vi "Green Board DC Bus Test.vi"(7 "HMP4040 Channel Settings":T1={"CH1 Voltage"=24.0, "CH1 Current"=1.0, "CH1 Output"=FALSE, "CH2 Voltage"=24.0, "CH2 Current"=3.0, "CH2 Output"=TRUE, "CH3 Voltage"=24.0, "CH3 Current"=1.0, "CH3 Output"=FALSE, "CH4 Voltage"=24.0, "CH4 Current"=1.0, "CH4 Output"=FALSE, "Master Output"=TRUE} {"CH4 Current" format="%.3f"; "CH4 Voltage" format="%.3f"; "CH3 Current" format="%.3f"; "CH3 Voltage" format="%.3f"; "CH2 Current" format="%.3f"; "CH2 Voltage" format="%.3f"; "CH1 Current" format="%.3f"; "CH1 Voltage" format="%.3f"}, 8 "error in (no error)":errorcluster, 9 "Board Selector":T2) -> (0 "error out":errorcluster, 2 "Message OUT":string, 3 "VISA Refnum out":refnum<visa-resource-name>, 5 "Pass/Fail":bool, 10 "Voltage DC charged":dbl, 11 "Voltage (0V)":dbl)   [LabVIEW 2022 SP3]
uses:
  Serial Board Com/Board Select.ctl
  HMP4000 Communication/HMP4040_ChannelControl.ctl
  Serial Board Com/ADCSelector GB.ctl
panel:
  in  "Message IN":string
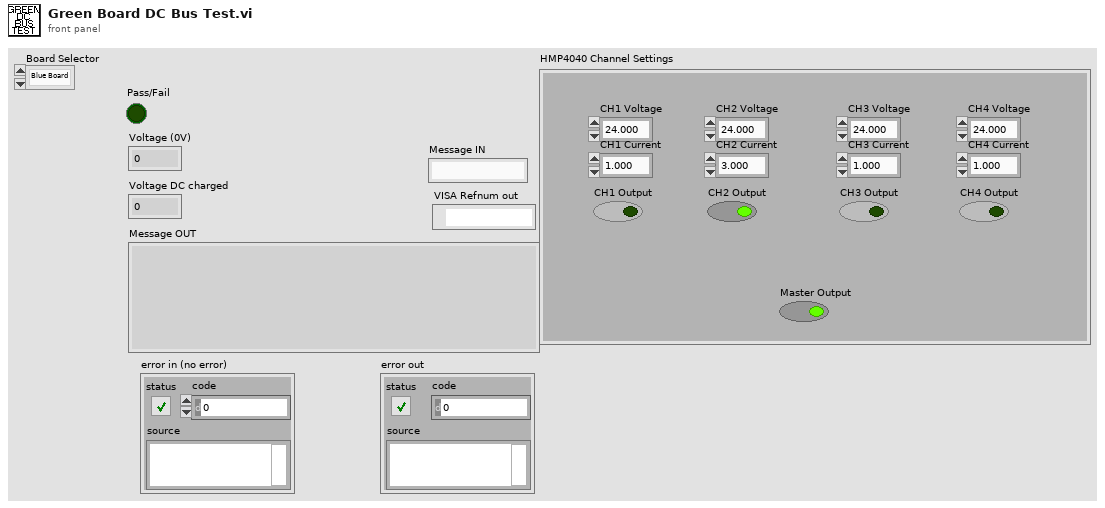
[diagram p1: front panel]
types:
  T1 = typedef "HMP4040_ChannelControl.ctl" = cluster{"CH1 Voltage":dbl, "CH1 Current":dbl, "CH1 Output":bool, "CH2 Voltage":dbl, "CH2 Current":dbl, "CH2 Output":bool, "CH3 Voltage":dbl, "CH3 Current":dbl, "CH3 Output":bool, "CH4 Voltage":dbl, "CH4 Current":dbl, "CH4 Output":bool, "Master Output":bool}
  T2 = typedef "Board Select.ctl" = enum16{"Blue Board", "Green Board"}
  T3 = typedef "ADCSelector GB.ctl" = enum16{"INVA_ISENSE_U", "INVA_ISENSE_V", "INVA_ISENSE_W", "INVA_UDC", "INVA_TEMP", "HB_ISENSE", "AUX_ISENSE_U", "AUX_ISENSE_V", "AUX_ISENSE_W", "VLINE_AB", "VLINE_BC", "VLINE_CA", "REF_1P5V", "VSENSE_POS_24V", "VSENSE_POS_5V", "VSENSE_NEG_15V", "TEST_POINT", "INVB_ISENSE_U", "INVB_ISENSE_V", "INVB_ISENSE_W", "INVB_UDC", "INVB_TEMP", "HB_TEMP", "AUXA_TEMP", "AUXB_TEMP", "AUXC_TEMP", "VOUT_AB", "VOUT_BC", "VOUT_CA", "REF_2P5V", "VSENSE_POS_15V", "VSENSE_POS_3P3V", "NET_ANALYZER"}
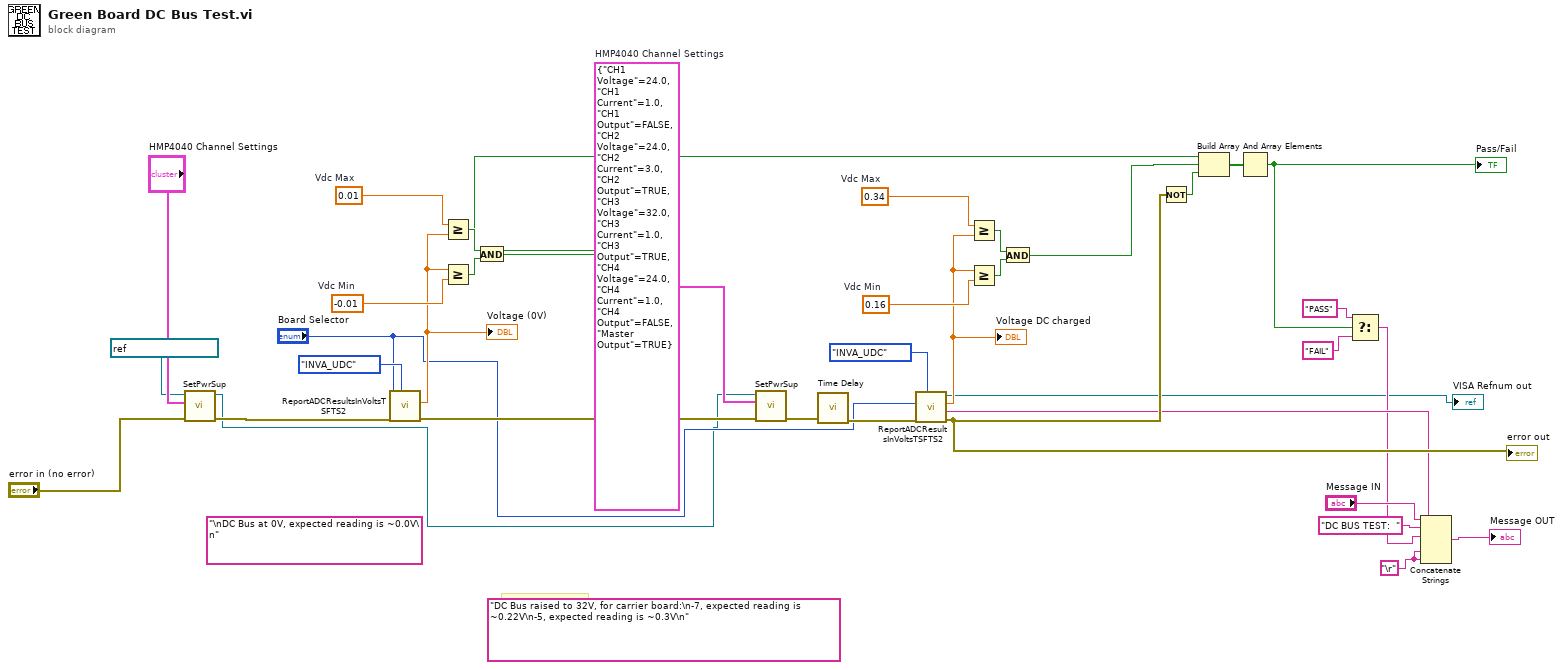
[diagram p0: block diagram]
diagram:
  w32 = T1 {"CH1 Voltage"=24.0, "CH1 Current"=1.0, "CH1 Output"=FALSE, "CH2 Voltage"=24.0, "CH2 Current"=3.0, "CH2 Output"=TRUE, "CH3 Voltage"=32.0, "CH3 Current"=1.0, "CH3 Output"=TRUE, "CH4 Voltage"=24.0, "CH4 Current"=1.0, "CH4 Output"=FALSE, "Master Output"=TRUE}  # HMP4040 Channel Settings
  (unwired) "DC Bus raised to 32V, for carrier board:\n-7, expected reading is ~0.22V\n-5, expected reading is ~0.3V\n"
  w14 = "\r"
  (unwired) "\nDC Bus at 0V, expected reading is ~0.0V\n"
  w27 = -0.01  # Vdc Min
  w26 = 0.01  # Vdc Max
  w35 = 0.16  # Vdc Min
  w36 = 0.34  # Vdc Max
  # "DC Bus == CH3"
  n1 = call "SetPwrSup.vi"("error in (no error)"="error in (no error)", "HMP4040 Channel Settings"="HMP4040 Channel Settings", "HMP4040 IN"=refnum<visa-resource-name> "HMP4040_FTS2" ("VISA resource name")) -> ("error out"=w9:errorcluster, "HMP4040_OUT"=w1:refnum<visa-resource-name>)  [unwired: 7 in]
  n2 = call "ReportADCResultsInVoltsTSFTS2.vi"("Green Board Enum"=ADCSelector_GB."INVA_UDC", "error in (no error)"=w9, "Board Selector"="Board Selector") -> ("error out"=w25:errorcluster, "Result"=w6:dbl)  [unwired: 5 in, 2 out]
  "Voltage (0V)" <- w6
  n3 = Greater Or Equal?(x=w26, y=w6) -> (x >= y?=w28:bool)
  n4 = Greater Or Equal?(x=w6, y=w27) -> (x >= y?=w29:bool)
  n5 = And(x=w28, y=w29) -> (x .and. y?=w12:bool)
  n6 = call "SetPwrSup.vi"("error in (no error)"=w25, "HMP4040 Channel Settings"=w32, "HMP4040 IN"=w1) -> ("error out"=w31:errorcluster)  [unwired: 7 in, 1 out]
  n7 = call "Time Delay"("error in (no error)"=w31) -> ("error out"=w30:errorcluster)  [unwired: 10 in]
  n8 = call "ReportADCResultsInVoltsTSFTS2.vi"("Green Board Enum"=ADCSelector_GB."INVA_UDC", "error in (no error)"=w30, "Board Selector"="Board Selector") -> ("error out"=w37:errorcluster, "Message OUT"=w22:string, "Result"=w5:dbl, "VISA Refnum out"=→"VISA Refnum out":refnum<visa-resource-name>)  [unwired: 5 in]
  "error out" <- w37
  "Voltage DC charged" <- w5
  n9 = Greater Or Equal?(x=w36, y=w5) -> (x >= y?=w34:bool)
  n10 = Greater Or Equal?(x=w5, y=w35) -> (x >= y?=w33:bool)
  n11 = And(x=w34, y=w33) -> (x .and. y?=w13:bool)
  n12 = Not(x=w37) -> (.not. x?=w24:bool)
  n13 = Build Array(w12, w13, w24) -> (w23:bool[])
  n14 = And Array Elements(Boolean array=w23) -> (logical AND=w16:bool)
  "Pass/Fail" <- w16
  n15 = Select(t="PASS", s=w16, f="FAIL") -> (s? t:f=w15:string)
  n16 = Concatenate Strings("Message IN", "DC BUS TEST:  " ("string"), w15, w22, w14, w14) -> (→"Message OUT":string)
